vi "script includes loader.vi"() -> ()   [LabVIEW 2013]
uses:
  <vilib>/NI/Tag Bus Module Framework/plugin discovery singleton/class discovery singleton methods.ctl
  <vilib>/NI/Tag Bus Module Framework/root configuration/TBM configuration.lvclass
  <vilib>/NI/Tag Bus Data Framework/Framework Configuration Classes/platypus configuration/PLConfigurationSerializer.lvlib
  <vilib>/NI/Tag Bus Module Framework/plugin discovery singleton/class discovery singleton.lvlib
panel:
  in  "vi path (blank=new)":path
  in  "cfg file path":path
  out "error out":errorcluster
  in  "Plugin Search Paths":path[](array[path])
  in  "target":i32
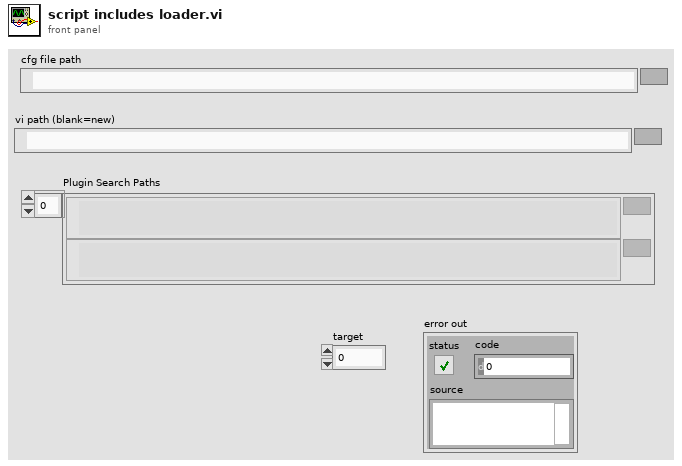
[diagram p1: front panel]
types:
  T1 = typedef "class discovery singleton.lvlib/class discovery singleton methods.ctl" = enum16{"add search paths", "load class by name", "list available classes", "get class path"}
  T2 = typedef "PLConfigurationSerializer.lvlib/file format.ctl" = cluster{"version":string, "data":string}
  T3 = typedef "PLConfigurationSerializer.lvlib/1_0_0_0 format.ctl" = cluster{"system":T4, "database":T7[]}
  T4 = typedef "PLConfigurationSerializer.lvlib/system hierarchy.ctl" = cluster{"system ID":string, "targets":T5[]}
  T5 = typedef "PLConfigurationSerializer.lvlib/target hierarchy.ctl" = cluster{"target ID":string, "engines":T6[]}
  T6 = typedef "PLConfigurationSerializer.lvlib/engine hierarchy.ctl" = cluster{"engine ID":string, "modules IDs":string[]}
  T7 = typedef "PLConfigurationSerializer.lvlib/configuration database.ctl" = cluster{"ID":string, "display name":string, "class":string, "version":string, "data":string}
  T8 = typedef "PLConfigurationSerializer.lvlib/targets cluster.ctl" = cluster{"Target Configuration":refnum<class "PL_Target Configuration.lvclass">, "engines":T9[]}
  T9 = typedef "PLConfigurationSerializer.lvlib/engines cluster.ctl" = cluster{"engine configuration":refnum<class "engine configuration.lvclass">, "modules":refnum<class "TBM module configuration.lvclass">[]}
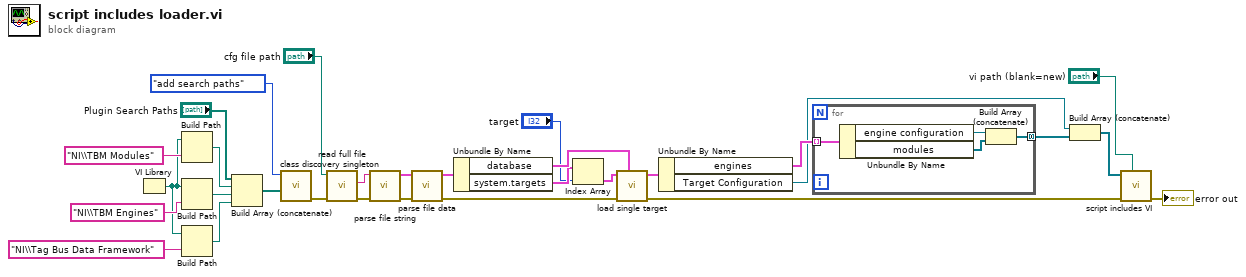
[diagram p0: block diagram]
diagram:
  n1 = VI Library() -> (path=w10:path)
  n2 = Build Path(base path=w10, name or relative path="NI\\TBM Modules") -> (appended path=w6:path)
  n3 = Build Path(base path=w10, name or relative path="NI\\TBM Engines") -> (appended path=w7:path)
  n4 = Build Path(base path=w10, name or relative path="NI\\Tag Bus Data Framework") -> (appended path=w8:path)
  n5 = Build Array (concatenate)("Plugin Search Paths", w6, w7, w8) -> (w4:path[])
  n6 = call <vilib>:"class discovery singleton.vi"("Plugin Search Paths"=w4, "method"=class_discovery_singleton_methods."add search paths") -> ("error out"=w18:errorcluster)  [unwired: 6 in, 3 out]
  n7 = call <vilib>:"read full file.vi"("error in"=w18, "file path"="cfg file path") -> ("error out"=w26:errorcluster, "data"=w27:string)  [unwired: 8 in]
  n8 = call <vilib>:"parse file string.vi"("error in"=w26, "data string"=w27) -> ("error out"=w28:errorcluster, "file format"=w29:T2)  [unwired: 8 in]
  n9 = call <vilib>:"parse file data.vi"("error in"=w28, "file format"=w29) -> ("error out"=w13:errorcluster, "file information"=w25:T3)  [unwired: 8 in]
  n10 = Unbundle By Name(w25) -> ("database"=w24:T7[], "system.targets"=w23:T5[])
  n11 = Index Array(array=w23, index="target") -> (element=w22:T5)
  n12 = call <vilib>:"load single target.vi"("database in"=w24, "error in"=w13, "target to load"=w22) -> ("error out"=w3:errorcluster, "targets cluster out"=w21:T8)  [unwired: 7 in]
  n13 = Unbundle By Name(w21) -> ("engines"=w17:T9[], "Target Configuration"=w15:refnum<class "PL_Target Configuration.lvclass">)
  n14 = for {
    tunnel: w17 -> [w34] mode=indexing
    tunnel: [w31] -> w16 mode=concatenating
    n15 = Unbundle By Name(w34) -> ("engine configuration"=w32:refnum<class "engine configuration.lvclass">, "modules"=w33:refnum<class "TBM module configuration.lvclass">[])
    n16 = Build Array (concatenate)(w32, w33) -> (w31:refnum<class "TBM configuration.lvclass">[])
  }
  n17 = Build Array (concatenate)(w15, w16) -> (w14:refnum<class "TBM configuration.lvclass">[])
  n18 = call "script includes VI.vi"("vi path (blank=new)"="vi path (blank=new)", "error in"=w3, "cfg objects"=w14) -> ("error out"=→"error out":errorcluster)  [unwired: 8 in]
